vi "SMU Adv Seq Step.vi"(8 "error in (no error)":errorcluster, 10 "JSONCluster":T1, 11 "IVI Refnum in":refnum<k15>) -> (0 "error out":errorcluster, 3 "IVI Refnum out":refnum<k15>)   [LabVIEW 2019, in "SupportVIs.lvlib"]
uses:
  SupportVIs.lvlib
  JSONCluster.ctl
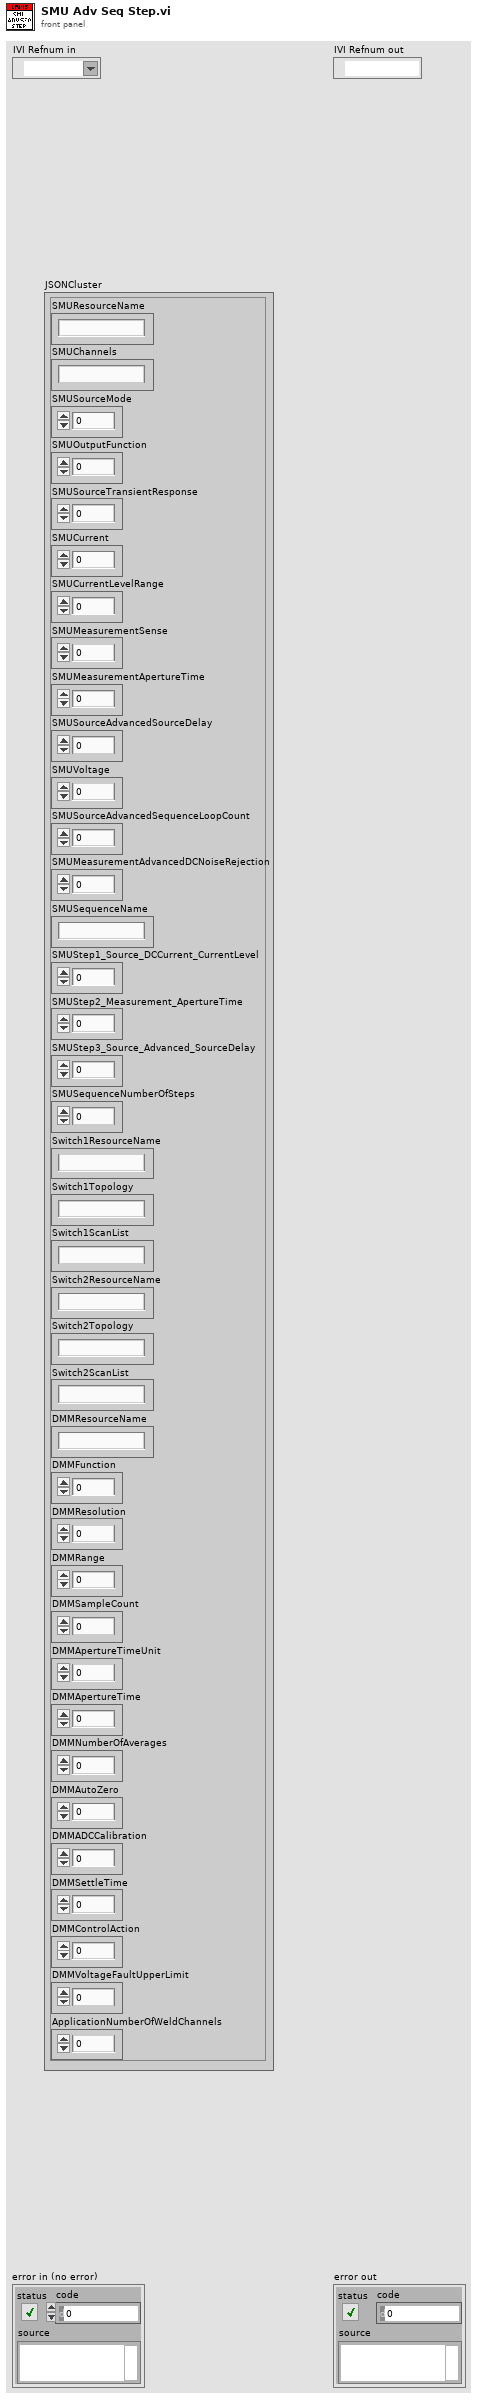
[diagram p1: front panel]
types:
  T1 = typedef "JSONCluster.ctl" = cluster{"SMUResourceName":string, "SMUChannels":string, "SMUSourceMode":i32, "SMUOutputFunction":i32, "SMUSourceTransientResponse":i32, "SMUCurrent":dbl, "SMUCurrentLevelRange":dbl, "SMUMeasurementSense":i32, "SMUMeasurementApertureTime":dbl, "SMUSourceAdvancedSourceDelay":dbl, "SMUVoltage":dbl, "SMUSourceAdvancedSequenceLoopCount":i32, "SMUMeasurementAdvancedDCNoiseRejection":i32, "SMUSequenceName":string, "SMUStep1_Source_DCCurrent_CurrentLevel":i32, "SMUStep2_Measurement_ApertureTime":i32, "SMUStep3_Source_Advanced_SourceDelay":i32, "SMUSequenceNumberOfSteps":i32, "Switch1ResourceName":string, "Switch1Topology":string, "Switch1ScanList":string, "Switch2ResourceName":string, "Switch2Topology":string, "Switch2ScanList":string, "DMMResourceName":string, "DMMFunction":i32, "DMMResolution":dbl, "DMMRange":dbl, "DMMSampleCount":i32, "DMMApertureTimeUnit":i32, "DMMApertureTime":dbl, "DMMNumberOfAverages":i32, "DMMAutoZero":i32, "DMMADCCalibration":i32, "DMMSettleTime":dbl, "DMMControlAction":i32, "DMMVoltageFaultUpperLimit":dbl, "ApplicationNumberOfWeldChannels":i32}
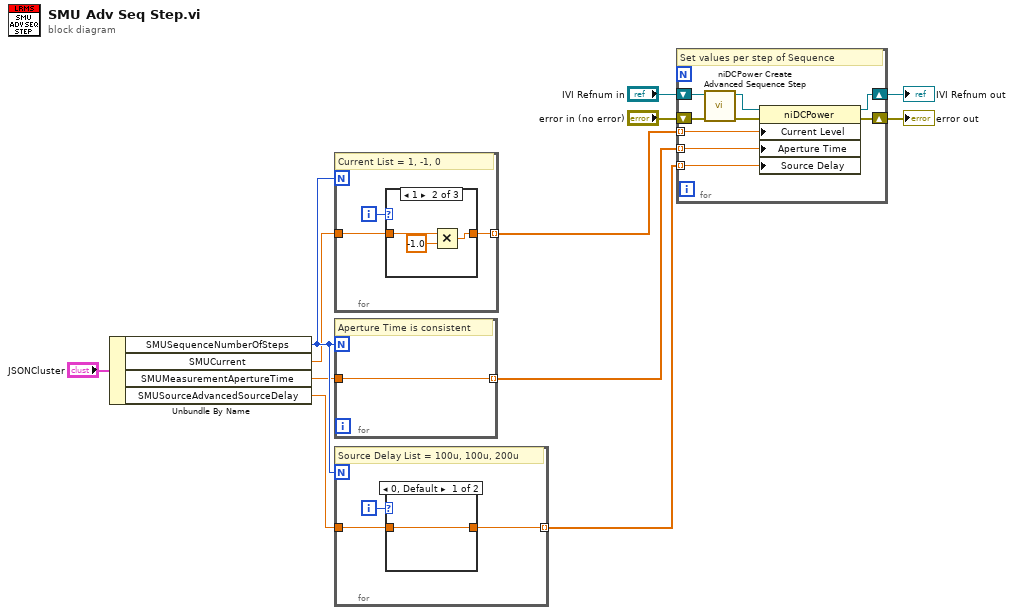
[diagram p0: block diagram]
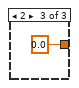
[diagram p3: hidden frame]
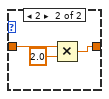
[diagram p4: hidden frame]
diagram:
  n1 = Unbundle By Name("JSONCluster") -> ("SMUSequenceNumberOfSteps"=w12:i32, "SMUCurrent"=w8:dbl, "SMUMeasurementApertureTime"=w9:dbl, "SMUSourceAdvancedSourceDelay"=w10:dbl)
  n2 = for {
    N: w12 -> [_]
    tunnel: w8 -> [w14]
    tunnel: [w13] -> w5 mode=indexing
    i -> [w15]
    # "Current List = 1, -1, 0"
    n3 = case shown="1" w15 {
      tunnel: w14 -> [w16 w18 _]
      tunnel: [w16 w19 0.0 ("current")] -> w13
      frame 0, Default {
      }
      frame 1 {
        n4 = Multiply(x=w18, y=-1.0) -> (x*y=w19:dbl)
      }
      frame 2 {
      }
    }
  }
  n5 = for {
    N: w12 -> [_]
    tunnel: w9 -> [w21]
    tunnel: [w21] -> w6 mode=indexing
    # "Aperture Time is consistent"
  }
  n6 = for {
    N: w12 -> [_]
    tunnel: w10 -> [w24]
    tunnel: [w23] -> w7 mode=indexing
    i -> [w22]
    # "Source Delay List = 100u, 100u, 200u"
    n7 = case shown="0, Default" w22 {
      tunnel: w24 -> [w25 w28]
      tunnel: [w25 w26] -> w23
      frame 0, Default {
      }
      frame 2 {
        n8 = Multiply(x=w28, y=2.0) -> (x*y=w26:dbl)
      }
    }
  }
  n9 = for {
    shift-right: [w34] -> w4
    shift-left: "error in (no error)" -> [w37]
    shift-right: [w33] -> w3
    shift-left: "IVI Refnum in" -> [w32]
    tunnel: w7 -> [w31] mode=indexing
    tunnel: w5 -> [w29] mode=indexing
    tunnel: w6 -> [w30] mode=indexing
    # "Set values per step of Sequence"
    n10 = call <instrlib>:"niDCPower Create Advanced Sequence Step.vi"("error in (no error)"=w37, "instrument handle"=w32) -> ("error out"=w35:errorcluster, "instrument handle out"=w36:refnum<k15>)  [unwired: 8 in]
    n11 = property class="niDCPower"(reference=w36, error in=w35, "Current Level"=w29, "Aperture Time"=w30, "Source Delay"=w31) -> (reference out=w33:refnum<k15>, error out=w34:errorcluster)
  }
  "error out" <- w4
  "IVI Refnum out" <- w3
